vi "Check for Invalid Char.vi"(1 "String":string, 2 "ASCII Num Value":i32) -> (0 "error out":errorcluster)   [LabVIEW 2012, in "FEM-03.lvlib"]
uses:
  FEM-03.lvlib
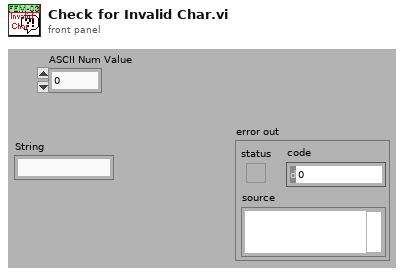
[diagram p1: front panel]
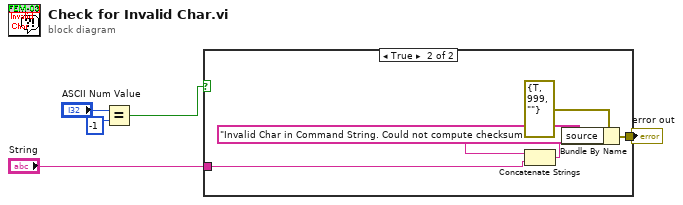
[diagram p0: block diagram]
diagram:
  n1 = Equal?(x="ASCII Num Value", y=-1) -> (x = y?=w2:bool)
  n2 = case shown="True" w2 {
    tunnel: [_ w6] -> w5
    tunnel: "String" -> [_ w10]
    frame False {
    }
    frame True {
      n3 = Concatenate Strings("Invalid Char in Command String. Could not compute checksum of " ("source"), w10) -> (w8:string)
      n4 = Bundle By Name(cluster=errorcluster {"status"=TRUE, "code"=999, "source"=""} ("error out"), "source"=w8) -> (w6:errorcluster)
    }
  }
  "error out" <- w5
